vi "Pump Action-Status Change Speeds.vi"(8 "error in (no error)":errorcluster, 10 "Message Data":variant, 11 "Data Cluster in":T1 {"Pump Info"."Direction" items=["CW", "CCW"]; "Pump Info"."Speed" format="%03.0f"}) -> (0 "error out":errorcluster, 3 "Data Cluster out":T1 {"Pump Info"."Direction" items=["CW", "CCW"]; "Pump Info"."Speed" format="%03.0f"})   [LabVIEW 2020, in "Pump.lvlib"]
uses:
  Pump.lvlib
  Pump Hardware Configuration.ctl
  support/Message Queue/Message Cluster.ctl
  support/HW Message Cluster.ctl
  support/Message Queue/Message Queue.lvlib
  <instrlib>/WM Pump/WM Pump.lvlib
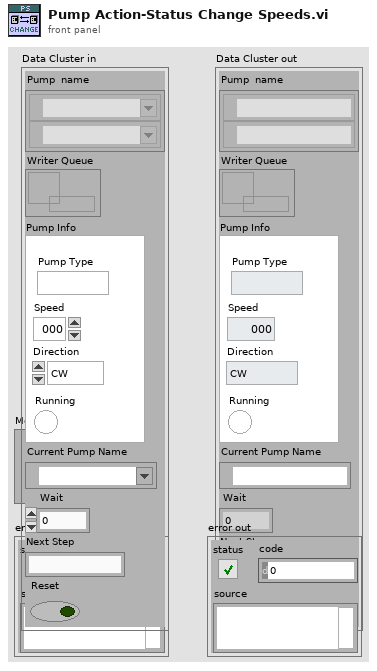
[diagram p1: front panel]
types:
  T1 = typedef "Pump.lvlib/Pump Hardware Configuration.ctl" = cluster{"Pump  name":refnum<visa-resource-name>[], "Writer Queue":refnum<queue>, "Pump Info":cluster{"Pump Type":string, "Speed":i32, "Direction":u16, "Running":bool}, "Current Pump Name":refnum<visa-resource-name>, "Wait":dbl, "Next Step":string, "Reset":bool}
  T2 = typedef "Message Queue.lvlib/HW Message Cluster.ctl" = cluster{"Writer Queue":refnum<queue>, "Writer Data":T3}
  T3 = typedef "Message Queue.lvlib/Message Cluster.ctl" = cluster{"Message":string, "Message Data":variant}
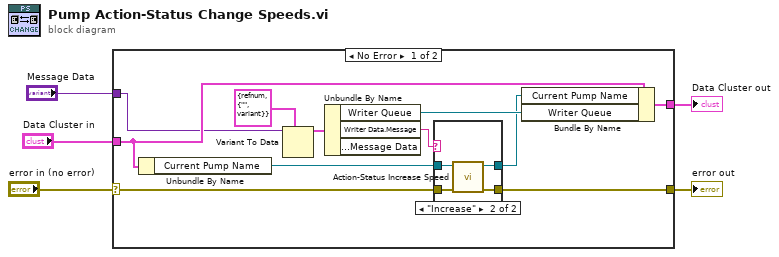
[diagram p0: block diagram]
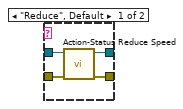
[diagram p2: hidden frame]
diagram:
  n1 = case shown="No Error" "error in (no error)" {
    selector: "error in (no error)" -> [w7 w25]
    tunnel: "Message Data" -> [w12 _]
    tunnel: [w16 w26] -> w4
    tunnel: "Data Cluster in" -> [w15 w26]
    tunnel: [w6 w25] -> w2
    frame No Error {
      n2 = Unbundle By Name(w15) -> ("Current Pump Name"=w9:refnum<visa-resource-name>)
      n3 = Variant To Data(type=T2 {"Writer Queue"=refnum, "Writer Data"={"Message"="", "Message Data"=variant}}, Variant=w12) -> (data=w13:T2)  [unwired: 1 in, 1 out]
      n4 = Unbundle By Name(w13) -> ("Writer Queue"=w11:refnum<queue>, "Writer Data.Message"=w10:string)  [unwired: 1 out]
      n5 = case shown="\"Increase\"" w10 {
        tunnel: w9 -> [w20 w24]
        tunnel: [w19 w23] -> w8
        tunnel: w7 -> [w18 w22]
        tunnel: [w17 w21] -> w6
        frame "Reduce", Default {
          n6 = call <instrlib>:"Action-Status Reduce Speed.vi"("error in (no error)"=w18, "VISA resource name"=w20) -> ("error out"=w17:errorcluster, "VISA resource name out"=w19:refnum<visa-resource-name>)  [unwired: 8 in]
        }
        frame "Increase" {
          n7 = call <instrlib>:"Action-Status Increase Speed.vi"("error in (no error)"=w22, "VISA resource name"=w24) -> ("error out"=w21:errorcluster, "VISA resource name out"=w23:refnum<visa-resource-name>)  [unwired: 8 in]
        }
      }
      n8 = Bundle By Name(cluster=w15, "Current Pump Name"=w8, "Writer Queue"=w11) -> (w16:T1)
    }
    frame Error {
    }
  }
  "Data Cluster out" <- w4
  "error out" <- w2
